vi "Force Off Limelight LED's.vi"(3 "error in":errorcluster) -> (10 "error out":errorcluster)   [LabVIEW 2018]
uses:
  <vilib>/Rock Robotics/Network Tables/NT Write Number.vi
panel:
  in  "Set LED":dbl=1.0
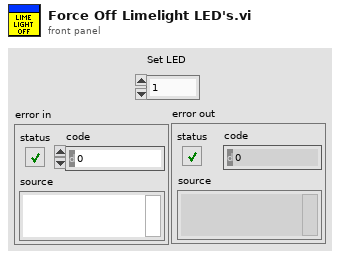
[diagram p1: front panel]
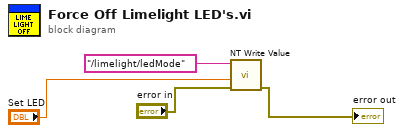
[diagram p0: block diagram]
diagram:
  n1 = call-poly <vilib>:"NT Write Value.vi"("error in"="error in", "Numeric"="Set LED", "Name"="/limelight/ledMode") -> ("error out"=→"error out":errorcluster)  [unwired: 8 in]
